vi "Example 2 - Local Bus Multiple Types.vi"() -> ()   [LabVIEW 2021]
uses:
  Omni-Bus/Omni_Bus.lvclass
  Omni-Bus/Support/Broad Types.ctl
  Local Bus/Local Bus.lvclass
  C:/Users/Tim/Documents/GitHub/Omni-Bus/Source/Omni-Bus/Bus Access/Bus_Access.lvclass
  <vilib>/Utility/Data Type/Type Definitions/Data Type.ctl
  Omni-Bus/Support/Write/Write DBL.vi
  Omni-Bus/Support/Write/Write String.vi
  Omni-Bus/Support/Write/Write Boolean.vi
  Omni-Bus/Support/Read/Read DBL.vi
  Omni-Bus/Support/Read/Read String.vi
  Omni-Bus/Support/Read/Read Boolean.vi
  <vilib>/TSA/Abstract Data Classes/Abs_Types/Double Float/Abs_Double Float.lvclass
  <vilib>/TSA/Abstract Data Classes/Abs_Types/String/Abs_String.lvclass
  <vilib>/TSA/Abstract Data Classes/Abs_Types/Boolean/Abs_Boolean.lvclass
  <vilib>/Utility/Data Type/NI_Data Type.lvlib
panel:
  in  "Write Boolean Tag":string
  in  "Boolean":bool
  out "Write Boolean error":errorcluster
  in  "Write String Tag":string
  in  "String":string
  out "Write String error":errorcluster
  out "Read Bool Error":errorcluster
  out "Read String error":errorcluster
  out "Boolean":bool
  out "String":string
  in  "Read Bool Tag":string
  in  "Read String Tag":string
  out "Read DBL error":errorcluster
  out "Write DBL error":errorcluster
  in  "Double":dbl
  in  "Write DBL Tag":string
  in  "stop":bool
  out "Double":dbl format="%.2f"
  in  "Read DBL Tag":string
  out "error out":errorcluster
  out "All Tags":string[](array[string])
  # "Reading and writing\nthe wrote type or tag\ngenerates an error"
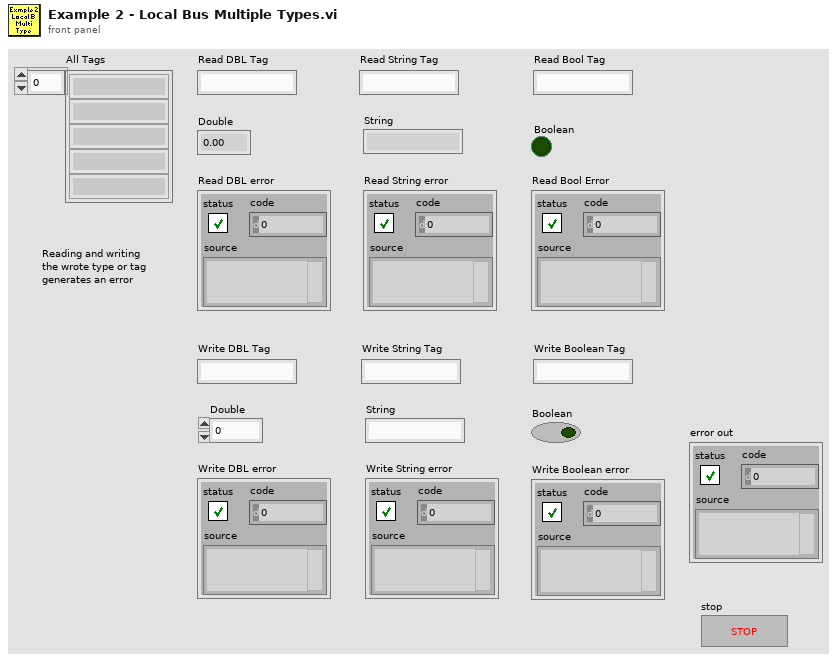
[diagram p1: front panel]
types:
  T1 = typedef "NI_Data Type.lvlib/Data Type.ctl" = enum8{"Invalid Type", "Void", "I8", "I16", "I32", "I64", "U8", "U16", "U32", "U64", "Single Float", "Double Float", "Extended Float", "Single Complex", "Double Complex", "Extended Complex", "Enum U8", "Enum U16", "Enum U32", "Enum U64", "Single Float With Unit", "Double Float With Unit", "Extended Float With Unit", "Single Complex with Unit", "Double Complex with Unit", "Extended Complex with Unit", "Boolean", "String", "Path", "Picture", "Tag", "Array", "Cluster", "Variant", "LV Variant", "Waveform", "Timestamp", "Digital Waveform", "Digital Data", "ExpressData", "Refnum", "External Data", "VI", "Poly VI", "LabVIEW Class Instance", "Fixed Point", "Set Collection", "Map Collection"}
  T2 = typedef "Omni_Bus.lvclass/Broad Types.ctl" = enum16{"All Tags", "NI Specific Type", "Boolean", "String", "Numeric", "Float", "Integer", "Collection", "All Value Types", "Non Value Types"}
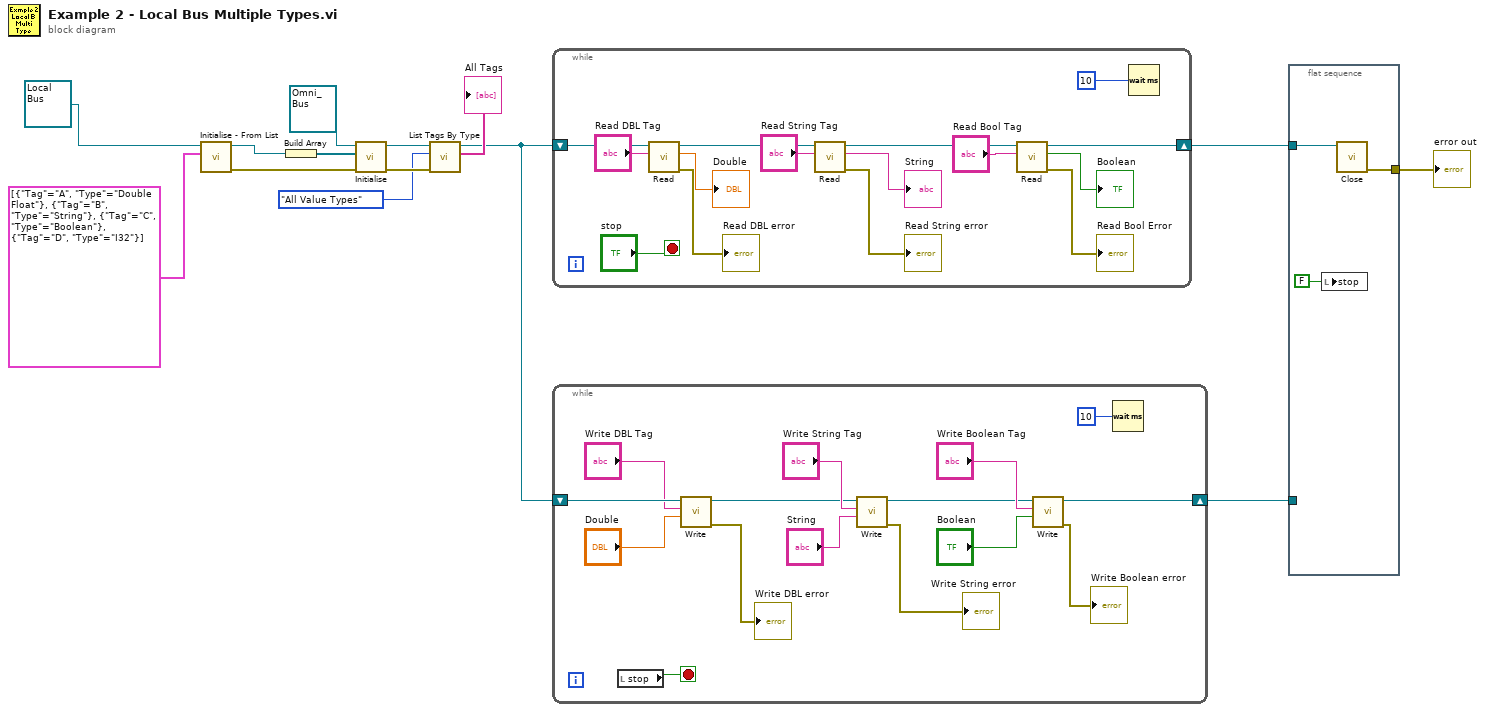
[diagram p0: block diagram]
diagram:
  n1 = call "Initialise - From List.vi"("Tag List"=cluster{"Tag":string, "Type":T1}[] [{"Tag"="A", "Type"=enum."Double Float"}, {"Tag"="B", "Type"=enum."String"}, {"Tag"="C", "Type"=enum."Boolean"}, {"Tag"="D", "Type"=enum."I32"}], "Local Bus in"=refnum<class "Local Bus.lvclass"> refnum ("Local Bus.lvclass")) -> ("error out"=w4:errorcluster, "Local Bus out"=w3:refnum<class "Local Bus.lvclass">)  [unwired: 8 in]
  n2 = Build Array(w3) -> (w13:refnum<class "Local Bus.lvclass">[])
  n3 = call-dynamic "Initialise.vi"("error in (no error)"=w4, "Bus Access"=w13, "Var Bus in"=refnum<class "Omni_Bus.lvclass"> refnum) -> ("error out"=w11:errorcluster, "Var Bus out"=w12:refnum<class "Omni_Bus.lvclass">)  [unwired: 7 in]
  n4 = call-dynamic "List Tags By Type.vi"("error in (no error)"=w11, "Broad Types"=Broad_Types."All Value Types", "Var Bus in"=w12) -> ("Tags"=→"All Tags":string[], "Var Bus out"=w6:refnum<class "Omni_Bus.lvclass">)  [unwired: 5 in, 2 out]
  n5 = while {
    shift-right: [w19] -> w7
    shift-left: w6 -> [w29]
    stop <- "stop" stop-if-true
    n6 = call-poly "Read.vi"("Tag"="Read DBL Tag", "Var Bus in"=w29) -> ("error out"=→"Read DBL error":errorcluster, "Numeric"=→"Double":dbl, "Var Bus out"=w22:refnum<class "Omni_Bus.lvclass">)  [unwired: 7 in]
    n7 = call-poly "Read.vi"("Tag"="Read String Tag", "Var Bus in"=w22) -> ("error out"=→"Read String error":errorcluster, "String"=→"String":string, "Var Bus out"=w20:refnum<class "Omni_Bus.lvclass">)  [unwired: 7 in]
    n8 = call-poly "Read.vi"("Tag"="Read Bool Tag", "Var Bus in"=w20) -> ("error out"=→"Read Bool Error":errorcluster, "Boolean"=→"Boolean":bool, "Var Bus out"=w19:refnum<class "Omni_Bus.lvclass">)  [unwired: 7 in]
    n9 = Wait (ms)(milliseconds to wait=u32 10) -> ()  [unwired: 1 out]
  }
  n10 = while {
    shift-right: [w30] -> w5
    shift-left: w6 -> [w44]
    stop <- w41 stop-if-true
    n11 = local read "stop"() -> (w41:bool)
    n12 = call-poly "Write.vi"("Numeric"="Double", "Tag"="Write DBL Tag", "Omni_Bus in"=w44) -> ("error out"=→"Write DBL error":errorcluster, "Omni_Bus out"=w35:refnum<class "Omni_Bus.lvclass">)  [unwired: 7 in]
    n13 = call-poly "Write.vi"("String"="String", "Tag"="Write String Tag", "Omni_Bus in"=w35) -> ("error out"=→"Write String error":errorcluster, "Omni_Bus out"=w31:refnum<class "Omni_Bus.lvclass">)  [unwired: 7 in]
    n14 = call-poly "Write.vi"("Boolean"="Boolean", "Tag"="Write Boolean Tag", "Omni_Bus in"=w31) -> ("error out"=→"Write Boolean error":errorcluster, "Omni_Bus out"=w30:refnum<class "Omni_Bus.lvclass">)  [unwired: 7 in]
    n15 = Wait (ms)(milliseconds to wait=u32 10) -> ()  [unwired: 1 out]
  }
  n16 = flat-sequence {
    tunnel: [w47] -> w8
    tunnel: w7 -> [w46]
    tunnel: w5 -> [_]
    frame #0 {
      n17 = local write "stop"(FALSE ("stop")) -> ()
      n18 = call-dynamic "Close.vi"("Data in"=w46) -> ("error out"=w47:errorcluster)  [unwired: 9 in, 1 out]
    }
  }
  "error out" <- w8
